vi "Copy and WireTagged Element.vi"(4 "Get All Objects? (F) In":bool, 6 "Delete Script Structure? (F) In":bool, 7 "Template Tag Details In":cluster{"Name":string, "Value":string}={"Name"="phygbuTag", "Value"="script"}, 8 "Error In":errorcluster, 9 "Template Refnum In":refnum<vi>, 10 "Terms In":T1[](array[typedef]), 11 "Diagram In":refnum<vi>) -> (0 "Error Out":errorcluster, 2 "All Objects Out":refnum<vi>[](array[refnum]), 3 "Diagram Out":refnum<vi>, 5 "TagName Out":string="phygbuTag")   [LabVIEW 2012, in "Scripting Tools.lvlib" / "XNode Support.lvlib"]
doc: "Searches the Template vi for a structure with a tag name and value given in Template Tag Details In and copies it to the Diagram and wires up as many terminals as it can, optionally deleting the structure and returning references to all the remaining objects.\nBased on a vi contributed by Greg Sands"
uses:
  XNode Support.lvlib
  <vilib>/XNodeSupport/XNodeTermIDPair.ctl
  <vilib>/XNodeSupport/XNodeTermRef.ctl
  <vilib>/XNodeSupport/XNodeString.ctl
  <vilib>/Utility/miscctls.llb/LVPositionTypeDef.ctl
  Scripting Tools.lvlib
  <vilib>/XNodeSupport/NI_XNodeSupport.lvlib
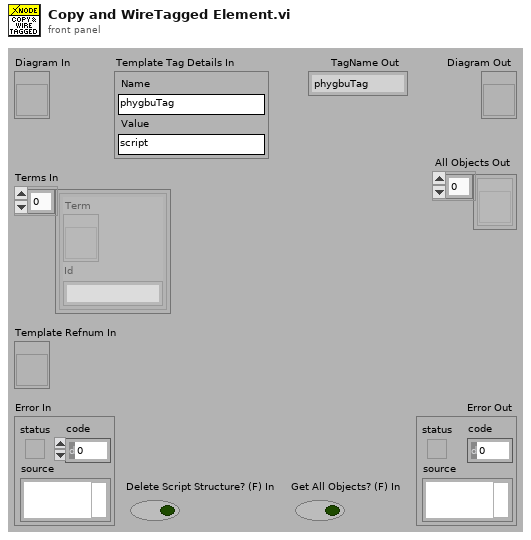
[diagram p1: front panel]
types:
  T1 = typedef "NI_XNodeSupport.lvlib/XNodeTermIDPair.ctl" = cluster{"Term":T2, "Id":T3}
  T2 = typedef "NI_XNodeSupport.lvlib/XNodeTermRef.ctl" = refnum<vi>
  T3 = typedef "NI_XNodeSupport.lvlib/XNodeString.ctl" = string
  T4 = typedef "LVPositionTypeDef.ctl" = cluster{"Left":i32, "Top":i32}
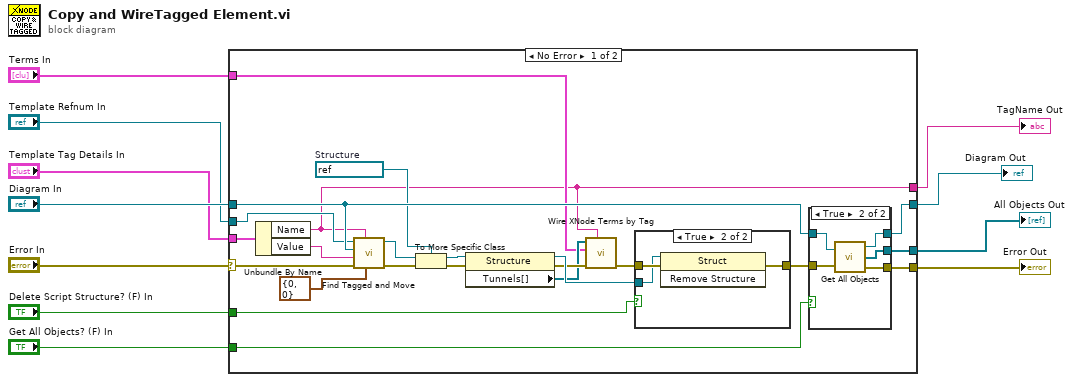
[diagram p0: block diagram]
diagram:
  n1 = case shown="No Error" "Error In" {
    selector: "Error In" -> [w20 w47]
    tunnel: [w34 w47] -> w11
    tunnel: [w33 _] -> w10
    tunnel: [w32 w46] -> w9
    tunnel: "Diagram In" -> [w31 w46]
    tunnel: "Delete Script Structure? (F) In" -> [w27 _]
    tunnel: "Template Refnum In" -> [w26 _]
    tunnel: "Terms In" -> [w16 _]
    tunnel: "Get All Objects? (F) In" -> [w15 _]
    tunnel: [w13 _] -> w2
    tunnel: "Template Tag Details In" -> [w14 _]
    frame No Error {
      w18 = refnum<vi> refnum  # Structure
      n2 = Unbundle By Name(w14) -> ("Name"=w13:string, "Value"=w12:string)
      n3 = call "Find Tagged and Move.vi"("position"=T4 {"Left"=0, "Top"=0}, "TagName"=w13, "error in"=w20, "TagValue"=w12, "Destination Diagram"=w31, "VI Refnum"=w26) -> ("error out"=w23:errorcluster, "Moved Tagged object"=w22:refnum<vi>)  [unwired: 4 out]
      n4 = To More Specific Class(target class=w18, reference=w22, error in=w23) -> (specific class reference=w17:refnum<vi>, error out=w24:errorcluster)
      n5 = property class="Structure"(reference=w17, error in=w24) -> (reference out=w29:refnum<vi>, error out=w25:errorcluster, "Tunnels[]"=w19:refnum<vi>[])
      n6 = call "Wire XNode Terms by Tag.vi"("TagName"=w13, "error in (no error)"=w25, "Term Refs"=w16, "Source References"=w19) -> ("error out"=w28:errorcluster)  [unwired: 7 out]
      n7 = case shown="True" w27 {
        tunnel: w28 -> [w42 w45]
        tunnel: w29 -> [_ w44]
        tunnel: [w42 w43] -> w30
        frame False {
        }
        frame True {
          n8 = invoke class="Struct" method="Remove Structure"(reference=w44, error in=w45) -> (error out=w43:errorcluster)  [unwired: 1 in, 2 out]
        }
      }
      n9 = case shown="True" w15 {
        tunnel: [w35 w41] -> w34
        tunnel: [_ w40] -> w33
        tunnel: [w36 w39] -> w32
        tunnel: w31 -> [w36 w38]
        tunnel: w30 -> [w35 w37]
        frame False {
        }
        frame True {
          n10 = call "Get All Objects.vi"("Diagram In"=w38, "error in"=w37) -> ("Diagram Out"=w39:refnum<vi>, "All Objects"=w40:refnum<vi>[], "error out"=w41:errorcluster)
        }
      }
    }
    frame Error {
    }
  }
  "Error Out" <- w11
  "All Objects Out" <- w10
  "Diagram Out" <- w9
  "TagName Out" <- w2
